vi "detectVarablesFromIP.vi"(3 "error in (no error)":errorcluster, 4 "PortIP":string, 5 "VISA resource name":refnum<visa-resource-name>="COM1" caption="端口号") -> (0 "error out":errorcluster, 1 "Data":T1[](array[typedef]), 2 "VISA resource name 2":refnum<visa-resource-name>="COM1" caption="端口号")   [LabVIEW 2010]
uses:
  OutputDataFormat.ctl
  GlobalCostants.vi
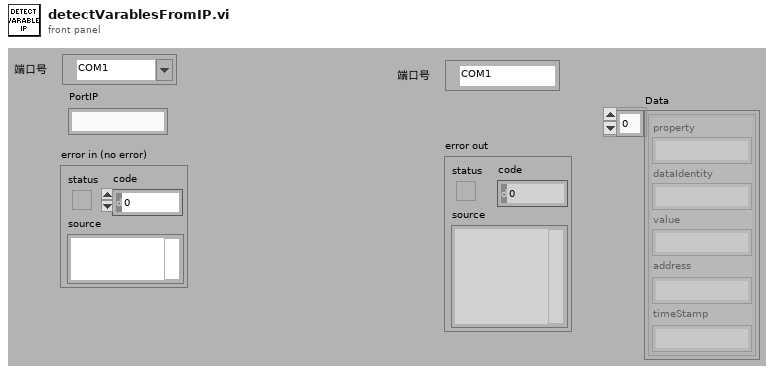
[diagram p1: front panel]
types:
  T1 = typedef "OutputDataFormat.ctl" = cluster{"property":string, "dataIdentity":string, "value":string, "address":string, "timeStamp":string}
  T2 = typedef "VarableStruct.ctl" = cluster{"Name":string, "StorageRefnum":refnum<file>, "Command":string, "IsDetecting":bool, "VarableID":T3}
  T3 = typedef "VarableID.ctl" = enum16{"current", "voltage", "power", "PF"}
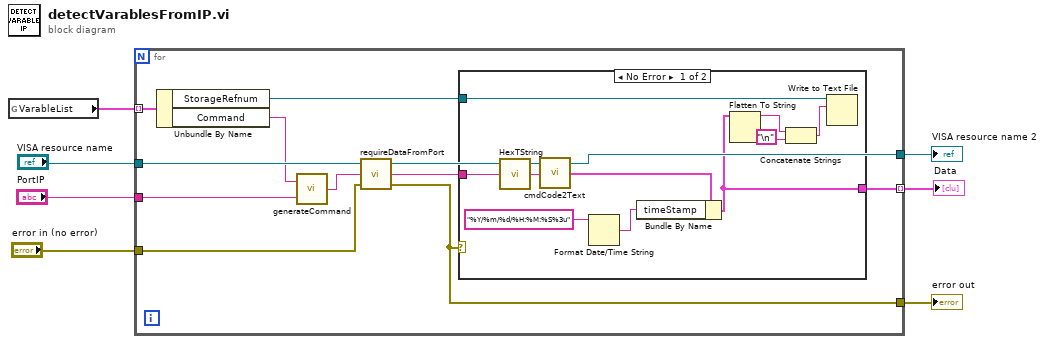
[diagram p0: block diagram]
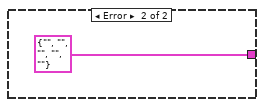
[diagram p2: hidden frame]
diagram:
  n1 = global read "GlobalCostants.vi" "VarableList"() -> (w7:T2[])
  n2 = for {
    tunnel: w7 -> [w15] mode=indexing
    tunnel: "VISA resource name" -> [w18]
    tunnel: [w17] -> w5
    tunnel: "error in (no error)" -> [w13]
    tunnel: [w12] -> w3
    tunnel: "PortIP" -> [w10]
    tunnel: [w8] -> w1 mode=indexing
    n3 = Unbundle By Name(w15) -> ("StorageRefnum"=w16:refnum<file>, "Command"=w11:string)
    n4 = call "generateCommand.vi"("IP"=w10, "CommandProtoType"=w11) -> ("Command"=w9:string)
    n5 = call "requireDataFromPort.vi"("error in (no error)"=w13, "Command"=w9, "VISA resource name"=w18) -> ("error out"=w12:errorcluster, "Data"=w14:string, "VISA resource name 2"=w17:refnum<visa-resource-name>)
    n6 = case shown="No Error" w12 {
      tunnel: w16 -> [w28 _]
      tunnel: w14 -> [w27 _]
      tunnel: [w22 T1 {"property"="", "dataIdentity"="", "value"="", "address"="", "timeStamp"=""} ("CommandText")] -> w8
      frame No Error {
        n7 = call "HexTString.vi"("input Hex"=w27) -> ("output string"=w26:string)
        n8 = call "cmdCode2Text.vi"("CommandCode"=w26) -> ("CommandText"=w21:T1)
        n9 = Format Date/Time String(time format string (%c)="%Y/%m/%d/%H:%M:%S%3u") -> (date/time string=w19:string)  [unwired: 2 in]
        n10 = Bundle By Name(cluster=w21, "timeStamp"=w19) -> (w22:T1)
        n11 = Flatten To String(anything=w22) -> (data string=w23:string)  [unwired: 3 in, 2 out]
        n12 = Concatenate Strings(w23, "\n") -> (w24:string)
        n13 = Write to Text File(file (use dialog)=w28, text=w24) -> ()  [unwired: 2 in, 3 out]
      }
      frame Error {
      }
    }
  }
  "VISA resource name 2" <- w5
  "error out" <- w3
  "Data" <- w1
